vi "Dresser DXD Close.vi"(0 "VISA session":refnum<visa-resource-name>, 11 "Error In (no error)":errorcluster) -> (15 "Error Out":errorcluster)   [LabVIEW 2015]
doc: "This VI closes the I/O interface with the Dresser DXD Series pressure transducer referenced by the VISA session.\n\nWritten by:\nBLOOMY CONTROLS, INC\nWINDSOR, CT 06095, USA\n860-298-9925\nwww.bloomy.com\nV2.0.0\nMay, 2002"
panel:
  # "For instructions on the use of this VI, press Ctrl+H to display the help window and move the mouse over the icon, controls, and indicators"
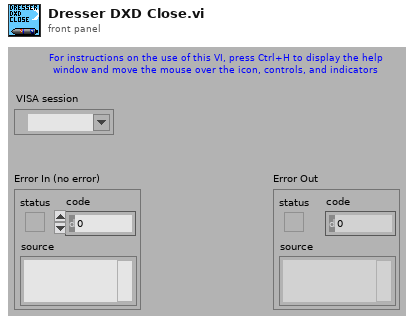
[diagram p1: front panel]
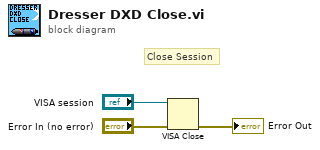
[diagram p0: block diagram]
diagram:
  # "Close Session"
  n1 = VISA Close(VISA resource name="VISA session", error in (no error)="Error In (no error)") -> (error out=→"Error Out":errorcluster)
